vi "5. Informative Queue Based Traffic Light Simulator.vi"() -> ()   [LabVIEW 2018]
uses:
  Typedefs/Traffic Light States for Queue based example.ctl
panel:
  out "Queue elements":cluster{"Next State":T1, "Wait Time":u32}[](array[cluster])
  in  "stop":bool
  out "Yellow":bool
  out "Green":bool
  out "Red":bool
  out "Traffic Lights Picture":picture
  # "Traffic Light Graphic Vector by Vecteezy\n(https://www.vecteezy.com/free-vector/graphic)"
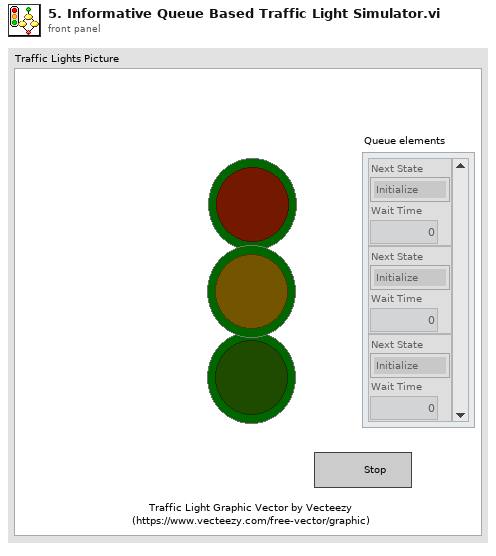
[diagram p1: front panel]
types:
  T1 = typedef "Traffic Light States for Queue based example.ctl" = enum16{"Initialize", "Red", "Yellow", "Green", "Wait", "Stop"}
  T2 = cluster{"Wait Before Red":u32, "Wait Before Yellow":u32, "Wait Before Green":u32}
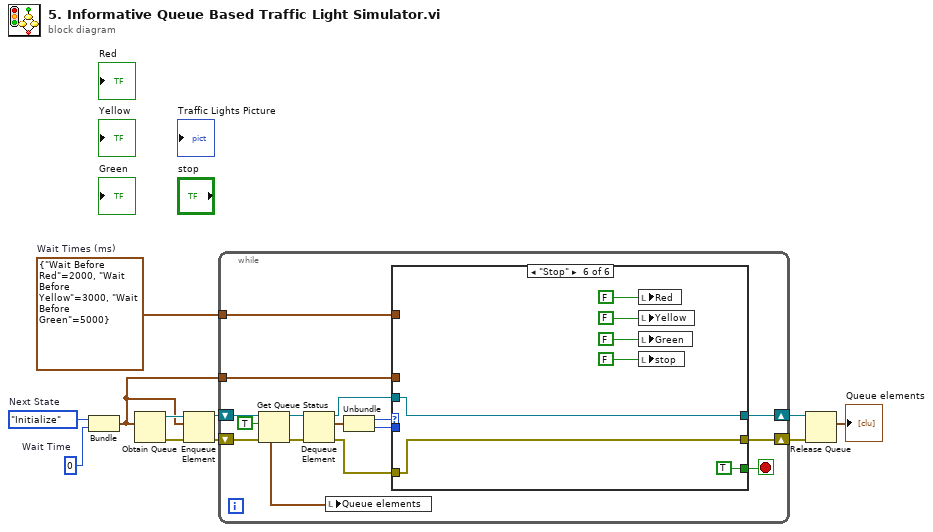
[diagram p0: block diagram]
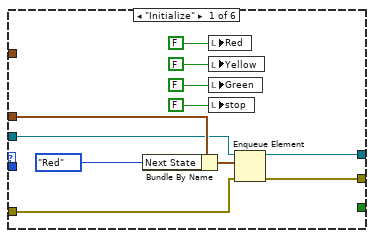
[diagram p2: hidden frame]
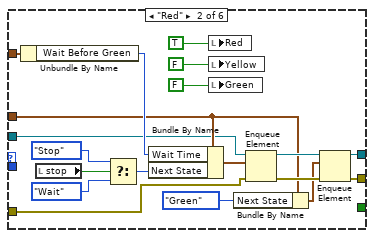
[diagram p3: hidden frame]
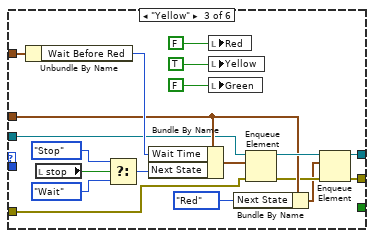
[diagram p4: hidden frame]
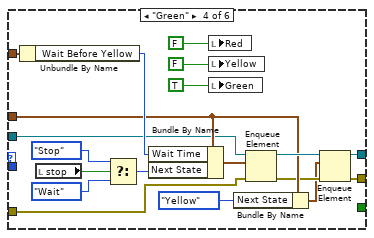
[diagram p5: hidden frame]
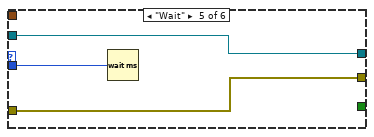
[diagram p6: hidden frame]
diagram:
  w9 = u32 0  # Wait Time
  w11 = T2 {"Wait Before Red"=2000, "Wait Before Yellow"=3000, "Wait Before Green"=5000}  # Wait Times (ms)
  w10 = Traffic_Light_States_for_Queue_based_example."Initialize"  # Next State
  n1 = Bundle("Next State"=w10, "Wait Time"=w9) -> (w5:cluster{"Next State":T1, "Wait Time":u32})  [unwired: 1 in]
  n2 = Obtain Queue(element data type=w5) -> (queue out=w8:refnum<queue>, error out=w6:errorcluster)  [unwired: 4 in, 1 out]
  n3 = Enqueue Element(queue=w8, element=w5, error in (no error)=w6) -> (queue out=w7:refnum<queue>, error out=w4:errorcluster)  [unwired: 1 in, 1 out]
  n4 = while {
    shift-right: [w22] -> w2
    shift-left: w7 -> [w15]
    tunnel: w11 -> [w27]
    tunnel: w5 -> [w23]
    shift-right: [w17] -> w3
    shift-left: w4 -> [w19]
    stop <- w26 stop-if-true
    n5 = Get Queue Status(queue=w15, return elements? (F)=TRUE, error in (no error)=w19) -> (queue out=w14:refnum<queue>, error out=w16:errorcluster, elements=w12:cluster{"Next State":T1, "Wait Time":u32}[])  [unwired: 5 out]
    n6 = Dequeue Element(queue=w14, error in (no error)=w16) -> (queue out=w21:refnum<queue>, element=w25:cluster{"Next State":T1, "Wait Time":u32}, error out=w18:errorcluster)  [unwired: 1 in, 1 out]
    n7 = local write "Queue elements"(w12) -> ()
    n8 = Unbundle(w25) -> ("Next State"=w24:T1, "Wait Time"=w20:u32)
    n9 = case shown="\"Stop\"" w24 {
      tunnel: [w31 w45 w65 w84 w98 w105] -> w22
      tunnel: w27 -> [_ w47 w67 w86 _ _]
      tunnel: [_ _ _ _ _ TRUE] -> w26
      tunnel: w23 -> [w34 w44 w64 w83 _ _]
      tunnel: w21 -> [w30 w41 w62 w81 w98 w105]
      tunnel: w20 -> [_ _ _ _ w97 _]
      tunnel: w18 -> [w29 w40 w61 w80 w96 w103]
      tunnel: [w28 w39 w58 w77 w96 w103] -> w17
      frame "Initialize" {
        n10 = Bundle By Name(cluster=w34, "Next State"=Traffic_Light_States_for_Queue_based_example."Red") -> (w32:cluster{"Next State":T1, "Wait Time":u32})
        n11 = local write "Red"(FALSE ("Red")) -> ()
        n12 = local write "Yellow"(FALSE ("Red")) -> ()
        n13 = local write "Green"(FALSE ("Red")) -> ()
        n14 = local write "stop"(FALSE ("stop")) -> ()
        n15 = Enqueue Element(queue=w30, element=w32, error in (no error)=w29) -> (queue out=w31:refnum<queue>, error out=w28:errorcluster)  [unwired: 1 in, 1 out]
      }
      frame "Red" {
        n16 = Unbundle By Name(w47) -> ("Wait Before Green"=w46:u32)
        n17 = local read "stop"() -> (w49:bool)
        n18 = Select(t=Traffic_Light_States_for_Queue_based_example."Stop" ("Next State"), s=w49, f=Traffic_Light_States_for_Queue_based_example."Wait" ("Next State")) -> (s? t:f=w50:T1)
        n19 = Bundle By Name(cluster=w44, "Wait Time"=w46, "Next State"=w50) -> (w53:cluster{"Next State":T1, "Wait Time":u32})
        n20 = local write "Red"(TRUE ("Red")) -> ()
        n21 = local write "Yellow"(FALSE ("Red")) -> ()
        n22 = local write "Green"(FALSE ("Red")) -> ()
        n23 = Bundle By Name(cluster=w44, "Next State"=Traffic_Light_States_for_Queue_based_example."Green") -> (w42:cluster{"Next State":T1, "Wait Time":u32})
        n24 = Enqueue Element(queue=w41, element=w53, error in (no error)=w40) -> (queue out=w52:refnum<queue>, error out=w57:errorcluster)  [unwired: 1 in, 1 out]
        n25 = Enqueue Element(queue=w52, element=w42, error in (no error)=w57) -> (queue out=w45:refnum<queue>, error out=w39:errorcluster)  [unwired: 1 in, 1 out]
      }
      frame "Yellow" {
        n26 = Unbundle By Name(w67) -> ("Wait Before Red"=w66:u32)
        n27 = local read "stop"() -> (w69:bool)
        n28 = Select(t=Traffic_Light_States_for_Queue_based_example."Stop" ("Next State"), s=w69, f=Traffic_Light_States_for_Queue_based_example."Wait" ("Next State")) -> (s? t:f=w70:T1)
        n29 = Bundle By Name(cluster=w64, "Wait Time"=w66, "Next State"=w70) -> (w73:cluster{"Next State":T1, "Wait Time":u32})
        n30 = local write "Red"(FALSE ("Red")) -> ()
        n31 = local write "Yellow"(TRUE ("Red")) -> ()
        n32 = local write "Green"(FALSE ("Red")) -> ()
        n33 = Bundle By Name(cluster=w64, "Next State"=Traffic_Light_States_for_Queue_based_example."Red") -> (w59:cluster{"Next State":T1, "Wait Time":u32})
        n34 = Enqueue Element(queue=w62, element=w73, error in (no error)=w61) -> (queue out=w72:refnum<queue>, error out=w60:errorcluster)  [unwired: 1 in, 1 out]
        n35 = Enqueue Element(queue=w72, element=w59, error in (no error)=w60) -> (queue out=w65:refnum<queue>, error out=w58:errorcluster)  [unwired: 1 in, 1 out]
      }
      frame "Green" {
        n36 = Unbundle By Name(w86) -> ("Wait Before Yellow"=w85:u32)
        n37 = local read "stop"() -> (w88:bool)
        n38 = Select(t=Traffic_Light_States_for_Queue_based_example."Stop" ("Next State"), s=w88, f=Traffic_Light_States_for_Queue_based_example."Wait" ("Next State")) -> (s? t:f=w89:T1)
        n39 = Bundle By Name(cluster=w83, "Wait Time"=w85, "Next State"=w89) -> (w92:cluster{"Next State":T1, "Wait Time":u32})
        n40 = local write "Red"(FALSE ("Red")) -> ()
        n41 = local write "Yellow"(FALSE ("Red")) -> ()
        n42 = local write "Green"(TRUE ("Red")) -> ()
        n43 = Bundle By Name(cluster=w83, "Next State"=Traffic_Light_States_for_Queue_based_example."Yellow") -> (w78:cluster{"Next State":T1, "Wait Time":u32})
        n44 = Enqueue Element(queue=w81, element=w92, error in (no error)=w80) -> (queue out=w91:refnum<queue>, error out=w79:errorcluster)  [unwired: 1 in, 1 out]
        n45 = Enqueue Element(queue=w91, element=w78, error in (no error)=w79) -> (queue out=w84:refnum<queue>, error out=w77:errorcluster)  [unwired: 1 in, 1 out]
      }
      frame "Wait" {
        n46 = Wait (ms)(milliseconds to wait=w97) -> ()  [unwired: 1 out]
      }
      frame "Stop" {
        n47 = local write "Red"(FALSE ("Red")) -> ()
        n48 = local write "Yellow"(FALSE ("Red")) -> ()
        n49 = local write "Green"(FALSE ("Red")) -> ()
        n50 = local write "stop"(FALSE ("stop")) -> ()
      }
    }
  }
  n51 = Release Queue(queue=w2, error in (no error)=w3) -> (remaining elements=→"Queue elements":cluster{"Next State":T1, "Wait Time":u32}[])  [unwired: 1 in, 2 out]
